vi "AE Data FGV.vi"(9 "AE":T2, 11 "Command":enum16{"Initialize", "Update", "Get"}(ring)) -> (1 "Index":i32, 3 "Array of AEs":T1=[{"Name"="Peng", "Go?"=TRUE, "Which batch?"=enum."Anything"}, {"Name"="Xue Sheng", "Go?"=TRUE, "Which batch?"=enum."Anything"}, {"Name"="Denny", "Go?"=TRUE, "Which batch?"=enum."Anything"}, {"Name"="Wilbur", "Go?"=TRUE, "Which batch?"=enum."Anything"}, {"Name"="Hafiz", "Go?"=TRUE, "Which batch?"=enum."Anything"}, {"Name"="James", "Go?"=TRUE, "Which batch?"=enum."Anything"}, {"Name"="Sharath", "Go?"=TRUE, "Which batch?"=enum."Anything"}, {"Name"="Habib", "Go?"=TRUE, "Which batch?"=enum."Anything"}, {"Name"="Stephen", "Go?"=TRUE, "Which batch?"=enum."Anything"}])   [LabVIEW 2016]
uses:
  AE Data.ctl
  Array AE Data.ctl
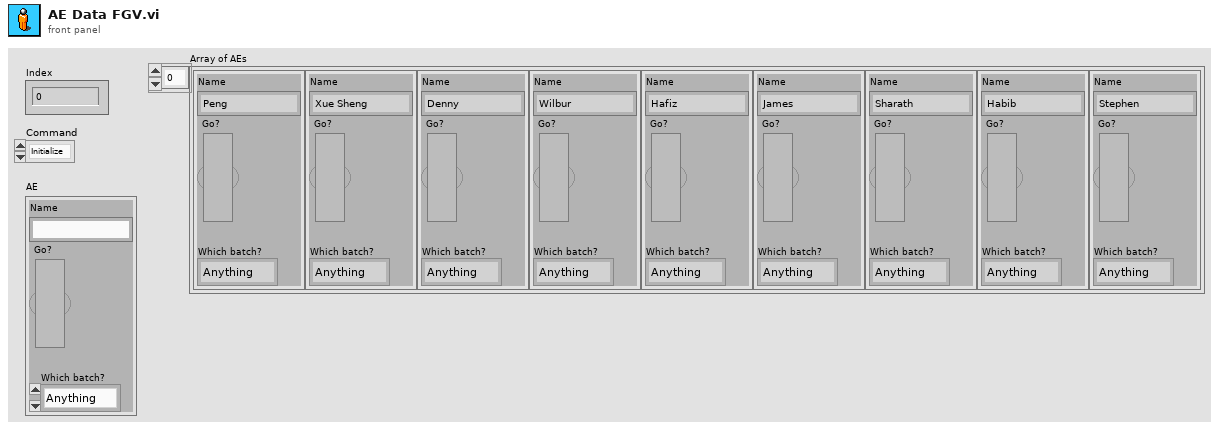
[diagram p1: front panel]
types:
  T1 = typedef "Array AE Data.ctl" = T2[]
  T2 = typedef "AE Data.ctl" = cluster{"Name":string, "Go?":bool, "Which batch?":enum16{"Anything", "First", "Second"}}
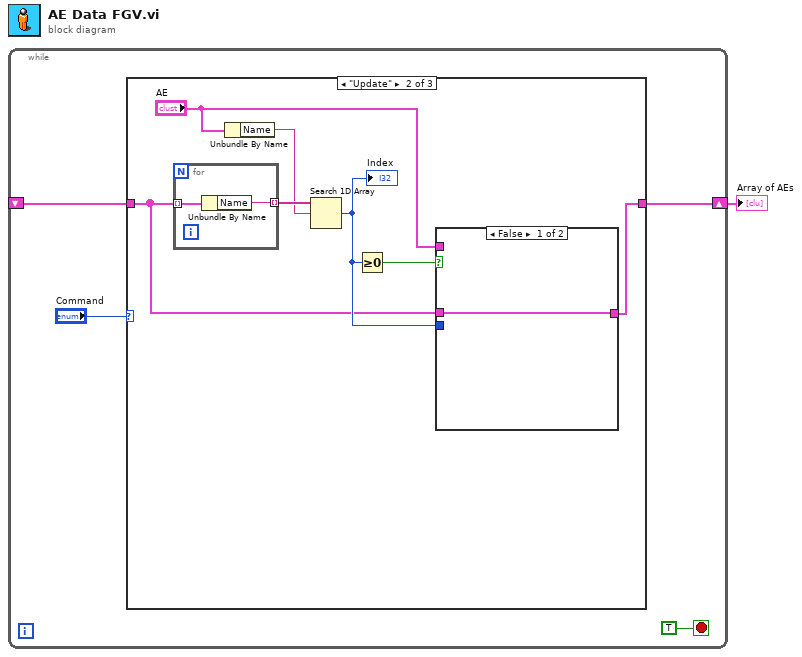
[diagram p0: block diagram]
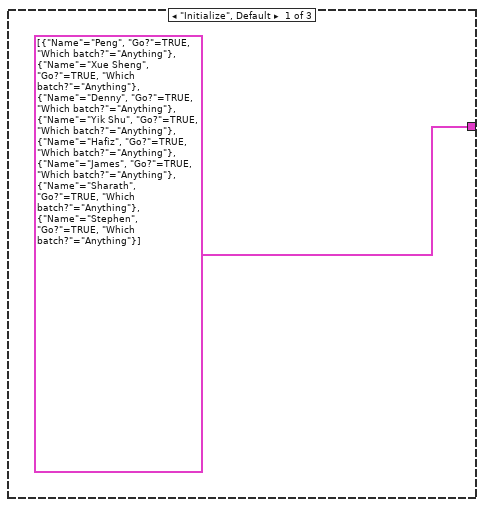
[diagram p2: hidden frame]
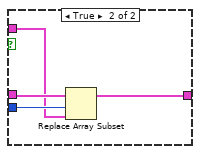
[diagram p3: hidden frame]
diagram:
  n1 = while {
    shift-right: [w3] -> w1
    shift-left: _ -> [w2]
    stop <- TRUE stop-if-true
    n2 = case shown="\"Update\"" "Command" {
      tunnel: [T1 [{"Name"="Peng", "Go?"=TRUE, "Which batch?"=enum."Anything"}, {"Name"="Xue Sheng", "Go?"=TRUE, "Which batch?"=enum."Anything"}, {"Name"="Denny", "Go?"=TRUE, "Which batch?"=enum."Anything"}, {"Name"="Yik Shu", "Go?"=TRUE, "Which batch?"=enum."Anything"}, {"Name"="Hafiz", "Go?"=TRUE, "Which batch?"=enum."Anything"}, {"Name"="James", "Go?"=TRUE, "Which batch?"=enum."Anything"}, {"Name"="Sharath", "Go?"=TRUE, "Which batch?"=enum."Anything"}, {"Name"="Stephen", "Go?"=TRUE, "Which batch?"=enum."Anything"}] ("Array of AEs") w7 w21] -> w3
      tunnel: w2 -> [_ w9 w21]
      frame "Initialize", Default {
      }
      frame "Update" {
        n3 = for {
          tunnel: w9 -> [w20] mode=indexing
          tunnel: [w19] -> w13 mode=indexing
          n4 = Unbundle By Name(w20) -> ("Name"=w19:string)
        }
        n5 = Unbundle By Name("AE") -> ("Name"=w12:string)
        n6 = Search 1D Array(1D array=w13, element=w12) -> (index of element=w10:i32)  [unwired: 1 in]
        "Index" <- w10
        n7 = Greater Or Equal To 0?(x=w10) -> (x >= 0?=w11:bool)
        n8 = case shown="False" w11 {
          tunnel: w10 -> [_ w18]
          tunnel: w9 -> [w14 w17]
          tunnel: "AE" -> [_ w16]
          tunnel: [w14 w15] -> w7
          frame False {
          }
          frame True {
            n9 = Replace Array Subset(array=w17, new element=w16, index=w18) -> (w15:T1)
          }
        }
      }
      frame "Get" {
      }
    }
  }
  "Array of AEs" <- w1
